vi "Get Header.vi"(8 "error in (no error)":errorcluster, 10 "header":string(combo)="User-Agent", 11 "HTTP Client Advanced in":refnum<class "HTTP Client Advanced.lvclass">) -> (0 "error out":errorcluster, 2 "value":string, 3 "HTTP Client Advanced out":refnum<class "HTTP Client Advanced.lvclass">)   [LabVIEW 2021, in "HTTP Client Advanced.lvclass"]
uses:
  HTTP Client Advanced.lvclass
  HTTP Client Advanced.lvclass/HTTP Client Advanced.ctl
  <vilib>/NI/Advanced HTTP Client/Session.lvclass
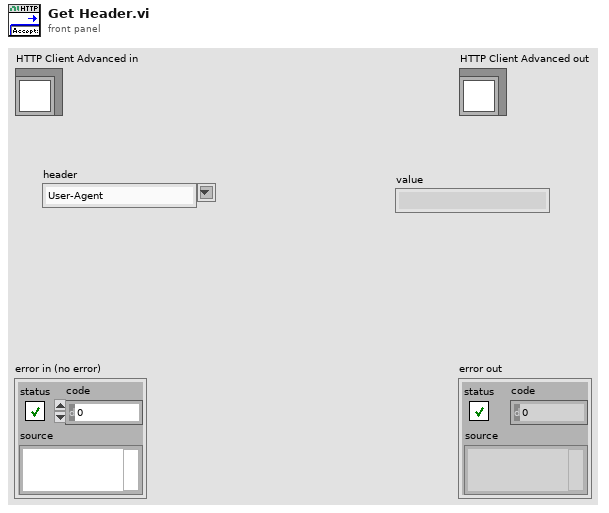
[diagram p1: front panel]
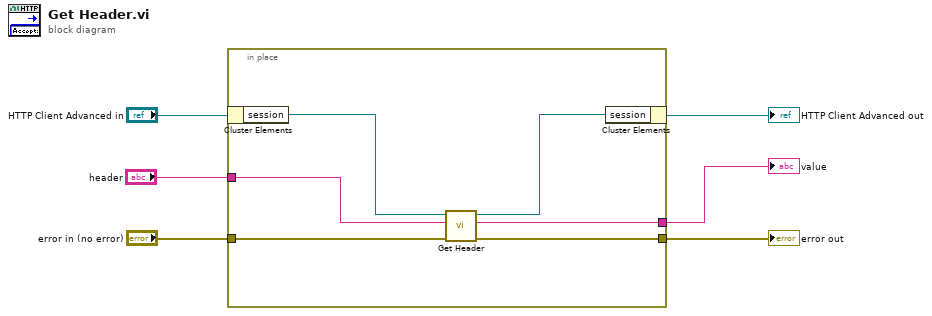
[diagram p0: block diagram]
diagram:
  n1 = in-place {
    in-place-border: "error in (no error)" -> [w12]
    in-place-border: [w11] -> w5
    in-place-border: "header" -> [w8]
    in-place-border: [w7] -> w1
    n2 = in-place-cluster #1("HTTP Client Advanced in") -> ("session"=w10:refnum<class "Session.lvclass">)
    n3 = call <vilib>:"Get Header.vi"("error in"=w12, "header"=w8, "session in"=w10) -> ("error out"=w11:errorcluster, "value"=w7:string, "session out"=w9:refnum<class "Session.lvclass">)  [unwired: 6 in]
    n4 = in-place-cluster #1("session"=w9) -> (→"HTTP Client Advanced out":refnum<class "HTTP Client Advanced.lvclass">)
  }
  "error out" <- w5
  "value" <- w1
